vi "GetSystemDefinitionPropertyValue_BinaryString.vi"(8 "error in (no error)":errorcluster, 10 "property name":string, 11 "BaseNodeType in":refnum<k24>) -> (0 "error out":errorcluster, 2 "value":string, 3 "BaseNodeType out":refnum<k24>)   [LabVIEW 2015, in "VeriStandTestUtilities.lvlib"]
uses:
  VeriStandTestUtilities.lvlib
  NationalInstruments.VeriStand.SystemStorage
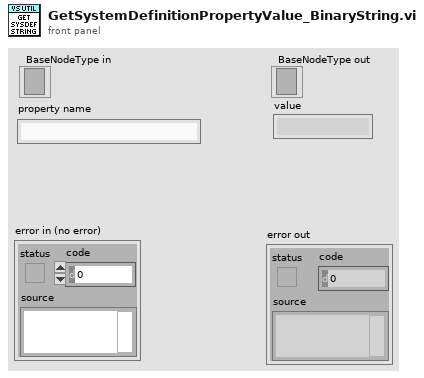
[diagram p1: front panel]
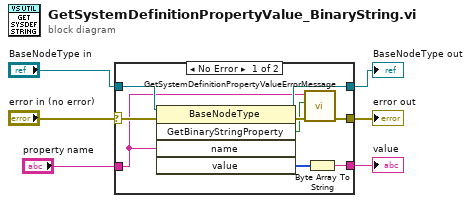
[diagram p0: block diagram]
diagram:
  n1 = case shown="No Error" "error in (no error)" {
    selector: "error in (no error)" -> [w14 w17]
    tunnel: "BaseNodeType in" -> [w15 w16]
    tunnel: "property name" -> [w9 _]
    tunnel: [w13 w16] -> w3
    tunnel: [w10 w17] -> w2
    tunnel: [w7 _] -> w1
    frame No Error {
      n2 = invoke class="BaseNodeType" method="GetBinaryStringProperty"(reference=w15, error in=w14, "name"=w9) -> (reference out=w13:refnum<k24>, error out=w11:errorcluster, "GetBinaryStringProperty"=w8:bool, "value"=w12:u8[])  [unwired: 2 in, 1 out]
      n3 = call "GetSystemDefinitionPropertyValueErrorMessage.vi"("error in (no error)"=w11, "successful?"=w8, "property name"=w9) -> ("error out"=w10:errorcluster)  [unwired: 8 in]
      n4 = Byte Array To String(unsigned byte array=w12) -> (string=w7:string)
    }
    frame Error {
    }
  }
  "error out" <- w2
  "BaseNodeType out" <- w3
  "value" <- w1
